vi "SMO.Dictionary.DeleteElement.vi"(6 "timeout (10ms)":i32=10, 8 "error in (no error)":errorcluster, 10 "Key":string, 11 "SMO.Dictionary":refnum<class "SMO.Dictionary.lvclass">) -> (0 "error out":errorcluster, 3 "SMO.Dictionary out":refnum<class "SMO.Dictionary.lvclass">, 4 "timed out?":bool)   [LabVIEW 2013, in "SMO.Dictionary.lvlib" / "SMO.Dictionary.lvclass"]
doc: "---------------------------------------------------------------\nJKI State Machine Objects™\nhttp://jki.net/state-machine-objects/\nCopyright (C) 2005-2015, JKI <info@jki.net>\nALL RIGHTS RESERVEDJKI State Machine Objects (SMO) 1.0.0.4\nJKI - JKI\nCopyright (c) 2015, JKI"
uses:
  SMO.Dictionary.lvclass
  Typedefs/PrivateEvents--SMO.Dictionary.KeyValue-Pair.ctl
  <vilib>/JKI/JKI SMO/SMO/SMO.lvclass
panel:
  # "For instructions on how to use the JKI State Machine Objects, examples and video tutorials, visit:\nhttp://jki.net/state-machine-objects/\n\nJKI State Machine Objects™\nhttp://jki.net/state-machine-objects/\nCopyright (C) 2005-2015, JKI <info@jki.net>\nALL RIGHTS RESERVED"
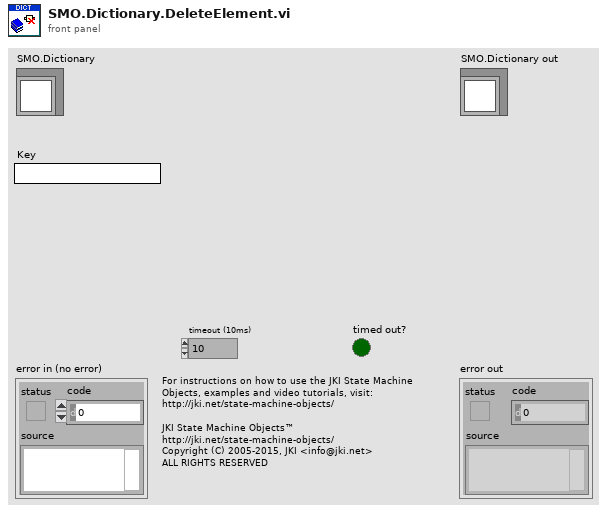
[diagram p1: front panel]
types:
  T1 = typedef "SMO.lvclass/SMOState --Enum.ctl" = enum16{"unknown", "Created", "Started", "Stopped"}
  T2 = typedef "SMO.Dictionary.lvlib/SMO.Dictionary.lvclass/PrivateEvents--SMO.Dictionary.KeyValue-Pair.ctl" = cluster{"Key":string, "Value":variant}
  T3 = typedef "SMO.Dictionary.lvlib/SMO.Dictionary.lvclass/PublicEvents--Cluster.ctl" = cluster{"Cleared":refnum<user-event>, "Deleted":refnum<user-event>, "Updated":refnum<user-event>}
  T4 = typedef "SMO.Dictionary.lvlib/SMO.Dictionary.lvclass/PrivateEvents--Cluster.ctl" = cluster{"Update":refnum<user-event>, "Clear Dictionary":refnum<user-event>, "Delete":refnum<user-event>, "Get":refnum<user-event>, "GetMultiple":refnum<user-event>}
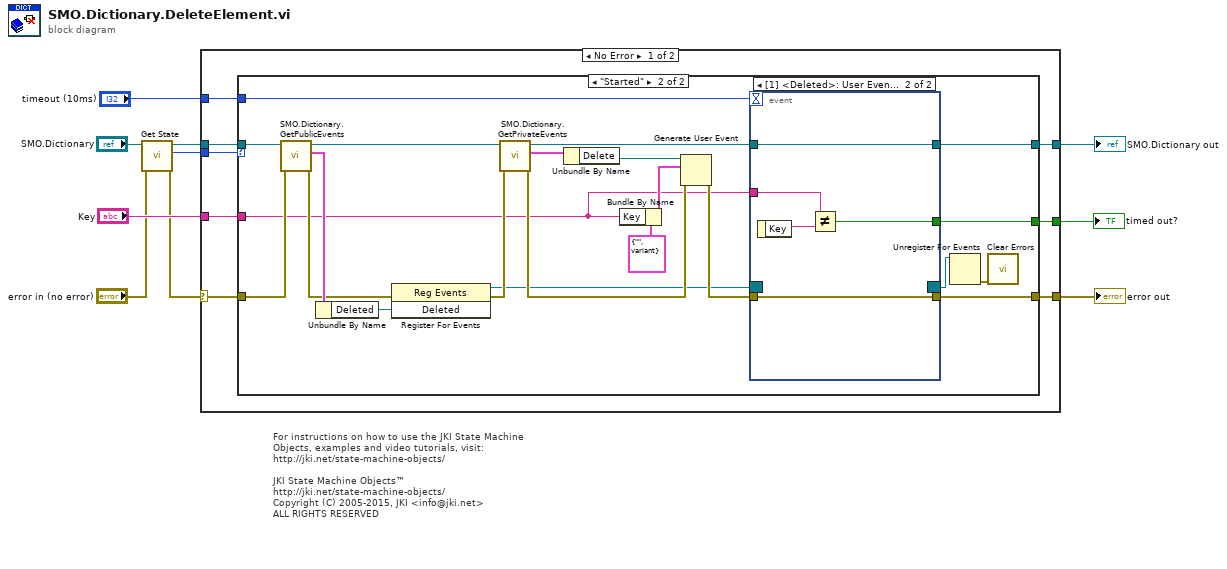
[diagram p0: block diagram]
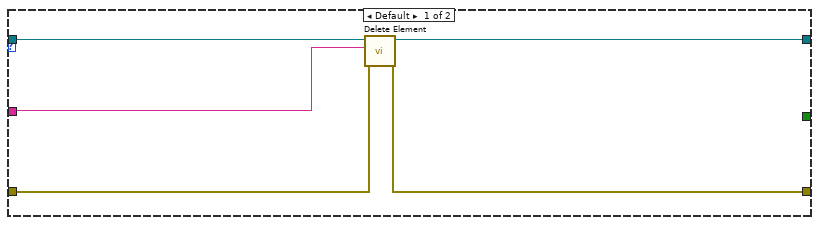
[diagram p2: hidden frame]
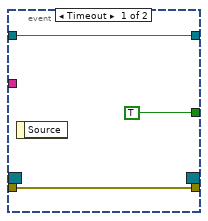
[diagram p3: hidden frame]
diagram:
  # "For instructions on how to use the JKI State Machine Objects, examples and video tutorials, visit:\nhttp://jki.net/state-machine-objects/\n\nJKI State Machine Objects™\nhttp://jki.net/state-machine-objects/\nCopyright (C) 2005-2015, JKI <info@jki.net>\nALL RIGHTS RESERVED"
  n1 = call <vilib>:"Get State.vi"("error in (no error)"="error in (no error)", "SMO"="SMO.Dictionary") -> ("error out"=w2:errorcluster, "SMO State"=w1:T1, "SMO out"=w4:refnum<class "SMO.Dictionary.lvclass">)  [unwired: 7 in]
  n2 = case shown="No Error" w2 {
    selector: w2 -> [w17 w55]
    tunnel: [w15 w55] -> w9
    tunnel: [w16 w54] -> w10
    tunnel: w4 -> [w18 w54]
    tunnel: "Key" -> [w12 _]
    tunnel: "timeout (10ms)" -> [w14 _]
    tunnel: [w13 _] -> w6
    tunnel: w1 -> [w11 _]
    frame No Error {
      n3 = case shown="\"Started\"" w11 {
        tunnel: w18 -> [w23 w39]
        tunnel: w17 -> [w21 w37]
        tunnel: [w19 w32] -> w16
        tunnel: [w20 w29] -> w15
        tunnel: w14 -> [_ w26]
        tunnel: [_ w25] -> w13
        tunnel: w12 -> [w22 w24]
        frame Default {
          n4 = call-dynamic "Delete Element.vi"("error in (no error)"=w21, "Key"=w22, "SMO.Dictionary in"=w23) -> ("error out"=w20:errorcluster, "SMO.Dictionary out"=w19:refnum<class "SMO.Dictionary.lvclass">)  [unwired: 6 in, 1 out]
        }
        frame "Started" {
          n5 = call "SMO.Dictionary.GetPublicEvents.vi"("error in (no error)"=w37, "SMO.Dictionary in"=w39) -> ("error out"=w36:errorcluster, "Public Events"=w40:T3, "SMO.Dictionary out"=w38:refnum<class "SMO.Dictionary.lvclass">)  [unwired: 7 in]
          n6 = Unbundle By Name(w40) -> ("Deleted"=w34:refnum<user-event>)
          n7 = register-events(error in=w36, w34) -> (reference out=w30:refnum<event-registration>, error out=w35:errorcluster)  [unwired: 1 in]
          n8 = call "SMO.Dictionary.GetPrivateEvents.vi"("error in (no error)"=w35, "SMO.Dictionary"=w38) -> ("error out"=w43:errorcluster, "Private Events"=w45:T4, "SMO.Dictionary out"=w33:refnum<class "SMO.Dictionary.lvclass">)  [unwired: 7 in]
          n9 = Unbundle By Name(w45) -> ("Delete"=w44:refnum<user-event>)
          n10 = Bundle By Name(cluster=T2 {"Key"="", "Value"=variant} ("Update"), "Key"=w24) -> (w42:T2)
          n11 = Generate User Event(user event=w44, event data cluster=w42, error in=w43) -> (error out=w31:errorcluster)  [unwired: 1 in, 1 out]
          n12 = event shown="[1] <Deleted>: User Event" {
            selector: w30 -> [_ _]
            dyn-events: [_ _] -> w28
            timeout: w26 -> [_ _]
            tunnel: w33 -> [w48 w53]
            tunnel: [w48 w53] -> w32
            tunnel: w31 -> [w47 w52]
            tunnel: [w47 w52] -> w29
            tunnel: [TRUE w49] -> w25
            tunnel: w24 -> [_ w50]
            event Timeout {
              n13 = event-data() -> ()  [unwired: 1 in, 1 out]
            }
            event User Event {
              n14 = event-data() -> ("Key"=w51:string)  [unwired: 1 in]
              n15 = Not Equal?(x=w50, y=w51) -> (x != y?=w49:bool)
            }
          }
          n16 = Unregister For Events(event registration refnum=w28) -> (error out=w27:errorcluster)  [unwired: 1 in]
          n17 = call <vilib>:"Clear Errors.vi"("error in (no error)"=w27) -> ()  [unwired: 6 in, 1 out]
        }
      }
    }
    frame Error {
    }
  }
  "error out" <- w9
  "SMO.Dictionary out" <- w10
  "timed out?" <- w6
